vi "Renishaw-XL80_SetMeasurementMode.vi"(8 "error in (no error)":errorcluster, 10 "MeasurementMode":i32(ring) items=["MEASUREMENT_INDETERMINATE", "MEASUREMENT_LINEAR_PLANE", "MEASUREMENT_LINEAR_RETRO", "MEASUREMENT_ANGULAR", "MEASUREMENT_STRAIGHTNESS_SHORT", "MEASUREMENT_STRAIGHTNESS_LONG", "MEASUREMENT_VELOCITY_RETRO"], 11 "Renishaw-XL80 in":refnum<class "Renishaw-XL80.lvclass">) -> (0 "error out":errorcluster, 3 "Renishaw-XL80 out":refnum<class "Renishaw-XL80.lvclass">)   [LabVIEW 2024, in "Renishaw-XL80.lvclass"]
doc: "MEASUREMENT_MODES\nThis enumerated type defines constants that specify the measurement mode.\n\nDefinition\n[v1_enum]typedef enum MEASUREMENT_MODES { MEASUREMENT_INDETERMINATE = 0, MEASUREMENT_LINEAR_PLANE = 1, MEASUREMENT_LINEAR_RETRO = 2, MEASUREMENT_ANGULAR = 3, MEASUREMENT_STRAIGHTNESS_SHORT = 4, MEASUREMENT_STRAIGHTNESS_LONG = 5} MEASUREMENT_MODES;\nComments\nThe v1_enum attribute indicates that the enumerated type will be transmitted as a 32-bit entity.\n\nMEASUREMENT_INDETERMINATE may be returned as part of the ML10 status. This would indicate that the ML10 is not responding. Attempting to use this value to set the measurement mode will fail. \nMEASUREMENT_LINEAR_PLANE indicates that the reading is treated as linear using a plane mirror. \nMEASUREMENT_LINEAR_RETRO indicates that the reading is treated as linear using a retro-reflector. \nMEASUREMENT_ANGULAR indicates that the reading is treated as angular. \nMEASUREMENT_STRAIGHTNESS_SHORT indicates that the reading is treated as straightness using short range optics. \nMEASUREMENT_STRAIGHTNESS_LONG indicates that the reading is treated as straightness using long range optics."
uses:
  Renishaw-XL80.lvclass
  Renishaw-XL80.lvclass/Renishaw-XL80.ctl
  D:/A.C.M/Example CSharp_64/bin/Debug/Interop.DX10SDKADAPTORLib.dll
  Example CSharp_64/bin/Debug/Interop.DX10SDKADAPTORLib.dll
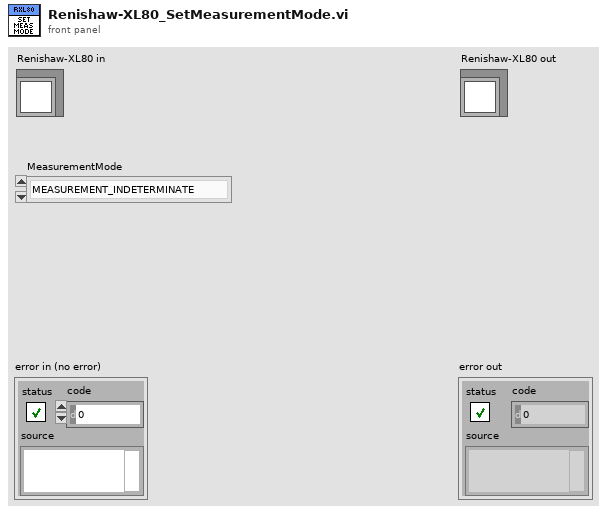
[diagram p1: front panel]
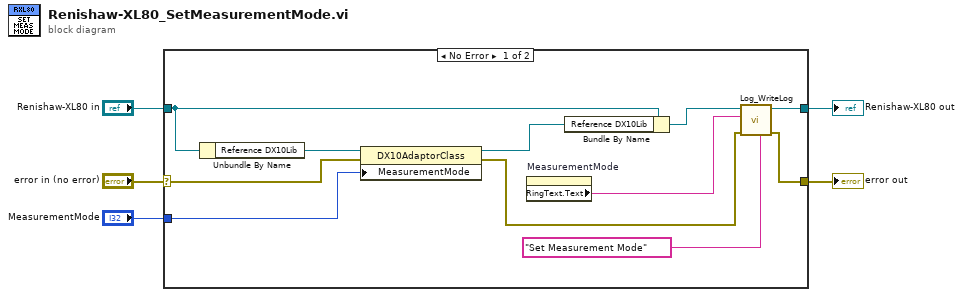
[diagram p0: block diagram]
diagram:
  n1 = case shown="No Error" "error in (no error)" {
    selector: "error in (no error)" -> [w13 w18]
    tunnel: [w8 w18] -> w4
    tunnel: [w10 w17] -> w2
    tunnel: "Renishaw-XL80 in" -> [w16 w17]
    tunnel: "MeasurementMode" -> [w12 _]
    frame No Error {
      n2 = Unbundle By Name(w16) -> ("Reference DX10Lib"=w15:refnum<k24>)
      n3 = property class="DX10AdaptorClass"(reference=w15, error in=w13, "MeasurementMode"=w12) -> (reference out=w14:refnum<k24>, error out=w6:errorcluster)
      n4 = property on="MeasurementMode" class="Ring (strict)"() -> ("RingText.Text"=w9:string)  [unwired: 2 in, 2 out]
      n5 = Bundle By Name(cluster=w16, "Reference DX10Lib"=w14) -> (w11:refnum<class "Renishaw-XL80.lvclass">)
      n6 = call-dynamic "Log_WriteLog.vi"("Additional text"="Set Measurement Mode", "error in (no error)"=w6, "Command"=w9, "Log in"=w11) -> ("error out"=w8:errorcluster, "Log out"=w10:refnum<class "Renishaw-XL80.lvclass">)  [unwired: 6 in]
    }
    frame Error {
    }
  }
  "error out" <- w4
  "Renishaw-XL80 out" <- w2
